vi "AuMT8852B EDR Rel Outp Pwr Summary Test.vi"() -> ()   [LabVIEW 2017]
doc: "This example shows how to extract Summary Test Results from the instrument. The Results panel will show a measurement summary of the test run. To view results from invividual test stages, use the Extended Test VIs."
panel:
  out "Results":T1 {"Peak 2DHx DPSK Absolute Power (dBm)" format="%.2f"; "Avg 2DHx DPSK Absolute Power (dBm)" format="%.2f"; "Min 2DHx DPSK Absolute Power (dBm)" format="%.2f"; "Max 2DHx DPSK Absolute Power (dBm)" format="%.2f"; "Peak 2DHx GFSK Absolute Power (dBm)" format="%.2f"; "Avg 2DHx GFSK Absolute Power (dBm)" format="%.2f"; "Min 2DHx GFSK Absolute Power (dBm)" format="%.2f"; "Max 2DHx GFSK Absolute Power (dBm)" format="%.2f"; "Peak 3DHx DPSK Absolute Power (dBm)" format="%.2f"; "Avg 3DHx DPSK Absolute Power (dBm)" format="%.2f"; "Min 3DHx DPSK Absolute Power (dBm)" format="%.2f"; "Max 3DHx DPSK Absolute Power (dBm)" format="%.2f"; "Peak 3DHx GFSK Absolute Power (dBm)" format="%.2f"; "Avg 3DHx GFSK Absolute Power (dBm)" format="%.2f"; "Min 3DHx GFSK Absolute Power (dBm)" format="%.2f"; "Max 3DHx GFSK Absolute Power (dBm)" format="%.2f"; "Avg power difference (dBm)" format="%.2f"; "Min power difference (dBm)" format="%.2f"; "Max power difference (dBm)" format="%.2f"; "Avg power difference (dBm)" format="%.2f"; "Min power difference (dBm)" format="%.2f"; "Max power difference (dBm)" format="%.2f"}
  in  "Settings":T2={"Low frequency selection"=enum."Use low frequency", "Medium frequency selection"=enum."Use medium frequency", "High frequency selection"=enum."Use high frequency", "Low TX frequency"=2480.0, "Low RX frequency"=2402.0, "Medium TX frequency"=2402.0, "Medium RX frequency"=2441.0, "High TX frequency"=2402.0, "High RX frequency"=2480.0, "Number of packets"=10, "PDPSK-PGFSK upper limit (dB) "=1.0, "PDPSK-PGFSK lower limit (dB)"=4.0, "2DHx test packet"=enum."Longest", "3DHx test packet"=enum."Longest", "Hop selection"=enum."Test with hopping off", "Test control"=enum."Loopback", "Hop mode"=enum."Defined", "Output Power Level"=enum."Max & Min"} {"PDPSK-PGFSK lower limit (dB)" format="%.2f"; "PDPSK-PGFSK upper limit (dB)" format="%.2f"}
  out "Addresses":string[](array[string])
  in  "Start/Stop (Start)":enum16{"Start", "Stop"}(ring)
  out "error out":errorcluster
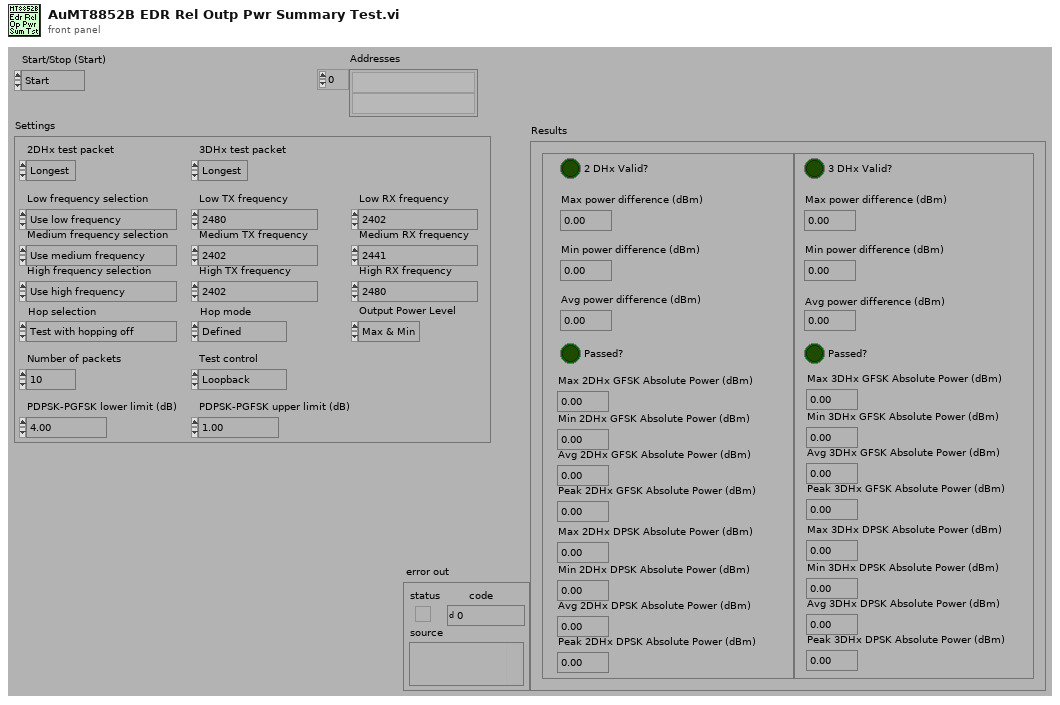
[diagram p1: front panel]
types:
  T1 = cluster{"2 DHx Valid?":bool, "Max power difference (dBm)":dbl, "Min power difference (dBm)":dbl, "Avg power difference (dBm)":dbl, "Passed?":bool, "3 DHx Valid?":bool, "Max power difference (dBm)":dbl, "Min power difference (dBm)":dbl, "Avg power difference (dBm)":dbl, "Passed?":bool, "Max 3DHx GFSK Absolute Power (dBm)":dbl, "Min 3DHx GFSK Absolute Power (dBm)":dbl, "Avg 3DHx GFSK Absolute Power (dBm)":dbl, "Peak 3DHx GFSK Absolute Power (dBm)":dbl, "Max 3DHx DPSK Absolute Power (dBm)":dbl, "Min 3DHx DPSK Absolute Power (dBm)":dbl, "Avg 3DHx DPSK Absolute Power (dBm)":dbl, "Peak 3DHx DPSK Absolute Power (dBm)":dbl, "Max 2DHx GFSK Absolute Power (dBm)":dbl, "Min 2DHx GFSK Absolute Power (dBm)":dbl, "Avg 2DHx GFSK Absolute Power (dBm)":dbl, "Peak 2DHx GFSK Absolute Power (dBm)":dbl, "Max 2DHx DPSK Absolute Power (dBm)":dbl, "Min 2DHx DPSK Absolute Power (dBm)":dbl, "Avg 2DHx DPSK Absolute Power (dBm)":dbl, "Peak 2DHx DPSK Absolute Power (dBm)":dbl}
  T2 = cluster{"Low frequency selection":enum16{"Don't use low frequency", "Use low frequency"}, "Medium frequency selection":enum16{"Don't use medium frequency", "Use medium frequency"}, "High frequency selection":enum16{"Don't use high frequency", "Use high frequency"}, "Low TX frequency":dbl, "Low RX frequency":dbl, "Medium TX frequency":dbl, "Medium RX frequency":dbl, "High TX frequency":dbl, "High RX frequency":dbl, "Number of packets":i32, "PDPSK-PGFSK upper limit (dB) ":dbl, "PDPSK-PGFSK lower limit (dB)":dbl, "2DHx test packet":enum16{"OFF", "Longest", "2-DH1", "2-DH3", "2-DH5"}, "3DHx test packet":enum16{"OFF", "Longest", "3-DH1", "3-DH3", "3-DH5"}, "Hop selection":enum16{"Test with hopping on", "Test with hopping off", "Test with hopping off and on"}, "Test control":enum16{"Loopback", "TX test"}, "Hop mode":enum16{"All", "Any", "Defined"}, "Output Power Level":enum16{"Min only", "Max only", "Max & Min"}}
  T3 = cluster{"Event status":enum16{"Event status disabled", "Event status enabled"}, "Message":enum16{"Message available disabled", "Message available enabled"}, "EUT Power State":u16, "State change":enum16{"State change disabled", "State change enabled"}, "Test failure":enum16{"Test failure disabled", "Test failure enabled"}, "Instrument status":enum16{"Instrument status disabled", "Instrument status enabled"}}
  T4 = cluster{"Completion":enum16{"Completion event disabled", "Completion event enabled"}, "Disconnect":enum16{"Disconnect event disabled", "Disconnect event enabled"}, "Connect":enum16{"Connect event disabled", "Connect event enabled"}, "Inquiry":enum16{"Inquiry event disabled", "Inquiry event enabled"}, "Temperature":enum16{"Temperature warning disabled", "Temperature warning enabled"}}
  T5 = cluster{"Reset":enum16{"Don't reset", "Reset"}, "Identity checking":enum16{"Don't query identity", "Query identity"}, "Simulation":enum16{"Don't simulate", "Simulate"}, "Range checking":enum16{"Don't check attribute ranges", "Check attribute ranges"}, "State caching":enum16{"Don't cache attributes", "Cache attributes"}, "Status checking":enum16{"Don't query instrument status", "Query instrument status"}}
  T6 = cluster{"Output power (Selected)":enum16{"Output power not selected", "Output power selected"}, "Power control (Selected)":enum16{"Power control not selected", "Power control selected"}, "Modulation index (Selected)":enum16{"Modulation index not selected", "Modulation index selected"}, "Initial carrier (Selected)":enum16{"Initial carrier not selected", "Initial carrier selected"}, "Carrier drift (Selected)":enum16{"Carrier drift not selected", "Carrier drift selected"}, "Single-slot sensitivity (Selected)":enum16{"Single-slot sensitivity not selected", "Single-slot sensitivity selected"}, "Multi-slot sensitivity (Selected)":enum16{"Multi-slot sensitivity not selected", "Multi-slot sensitivity selected"}, "Maximum input power (Selected)":enum16{"Maximum input power not selected", "Maximum input power selected"}, "Relative transmit power (Selected)":enum16{"Rel. transmit power not selected", "Rel. transmit power selected"}, "Carrier frequency stability and modulation (Selected)":enum16{"Carrier freq. and stability not selected", "Carrier freq. and stability selected"}, "Differential phase encoding":enum16{"Differential phase not selected", "Differential phase selected"}, "Sensitivity (Selected)":enum16{"Sensitivity not selected", "Sensitivity selected"}, "BER floor sensitivity (Selected)":enum16{"BER floor sensitivity not selected", "BER floor sensitivity selected"}, "EDR Maximum input power (Selected)":enum16{"EDR Max input power not selected", "EDR Max input power selected"}}
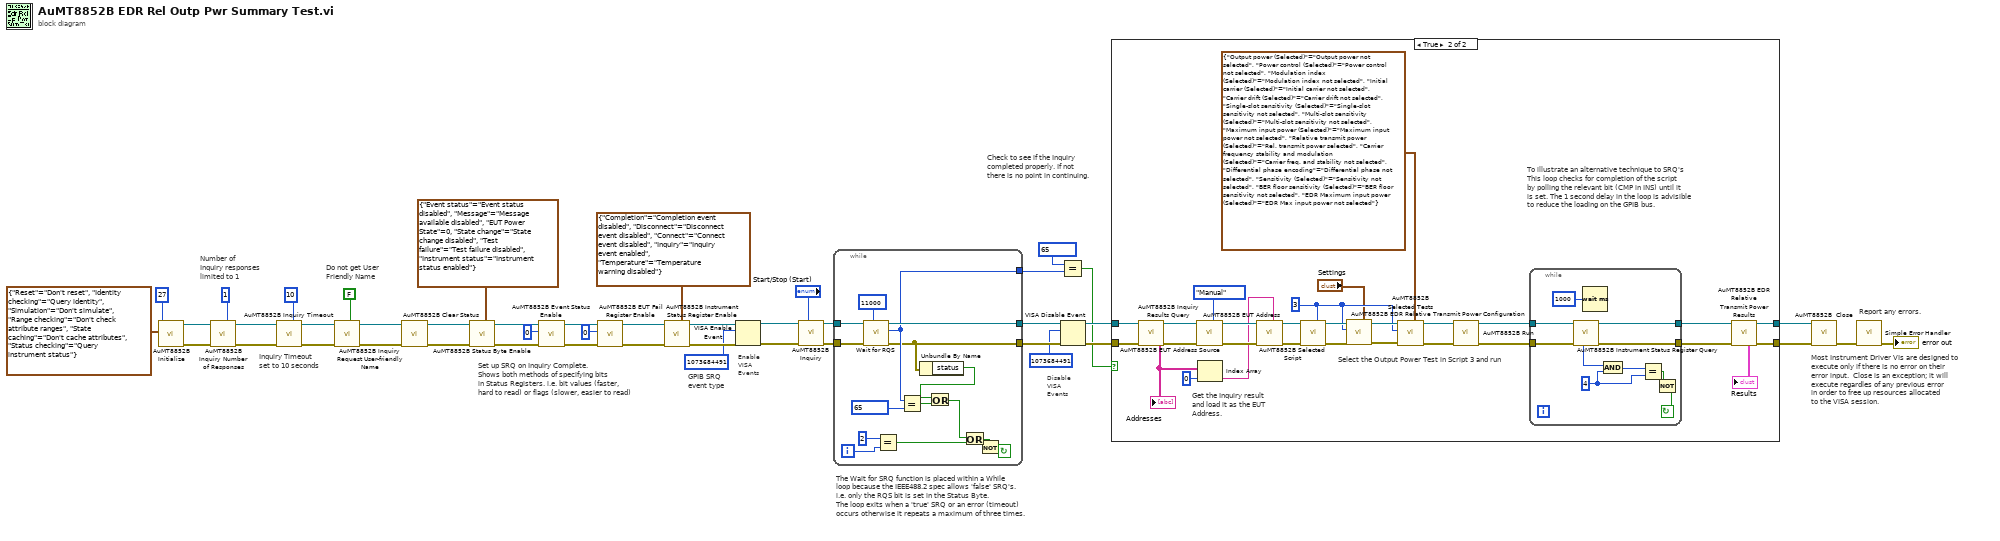
[diagram p0: block diagram]
diagram:
  # "Most Instrument Driver VIs are designed to\nexecute only if there is no error on their\nerror input.  Close is an exception; it will \nexecute regardles of any previous error\nin order to free up resources allocated\nto the VISA session."
  # "Report any errors."
  # "Check to see if the Inquiry\ncompleted properly. If not\nthere is no point in continuing."
  # "Disable\nVISA\nEvents"
  # "The Wait for SRQ function is placed within a While\nloop because the IEEE488.2 spec allows 'false' SRQ's.\ni.e. only the RQS bit is set in the Status Byte.\nThe loop exits when a 'true' SRQ or an error (timeout) \noccurs otherwise it repeats a maximum of three times."
  # "Enable\nVISA\nEvents"
  # "Set up SRQ on Inquiry Complete.\nShows both methods of specifying bits\nin Status Registers. i.e. bit values (faster, \nhard to read) or flags (slower, easier to read)"
  # "Inquiry Timeout\nset to 10 seconds"
  # "Number of\nInquiry responses\nlimited to 1"
  # "GPIB SRQ\nevent type"
  # "Do not get User\nFriendly Name"
  n1 = call <instrlib>:"AuMT8852B  Initialize.vi"("Options"=T5 {"Reset"=enum."Don't reset", "Identity checking"=enum."Query identity", "Simulation"=enum."Don't simulate", "Range checking"=enum."Don't check attribute ranges", "State caching"=enum."Don't cache attributes", "Status checking"=enum."Query instrument status"}, "GPIB Address (27)"=27) -> ("error out"=w43:errorcluster, "VISA session out"=w44:refnum<visa-resource-name>)  [unwired: 8 in]
  n2 = call <instrlib>:"AuMT8852B Inquiry Number of Responses.vi"("Responses (1)"=1, "error in (no error)"=w43, "VISA session"=w44) -> ("error out"=w41:errorcluster, "VISA session out"=w42:refnum<visa-resource-name>)  [unwired: 5 in, 2 out]
  n3 = call <instrlib>:"AuMT8852B Inquiry Timeout.vi"("Timeout (1)"=10, "error in (no error)"=w41, "VISA session"=w42) -> ("error out"=w38:errorcluster, "VISA session out"=w39:refnum<visa-resource-name>)  [unwired: 5 in, 2 out]
  n4 = call <instrlib>:"AuMT8852B Inquiry Request User-friendly Name.vi"("Status (T)"=FALSE, "error in (no error)"=w38, "VISA session"=w39) -> ("error out"=w33:errorcluster, "VISA session out"=w34:refnum<visa-resource-name>)  [unwired: 5 in, 2 out]
  n5 = call <instrlib>:"AuMT8852B Clear Status.vi"("error in (no error)"=w33, "VISA session"=w34) -> ("error out"=w31:errorcluster, "VISA session out"=w32:refnum<visa-resource-name>)  [unwired: 7 in, 1 out]
  n6 = call <instrlib>:"AuMT8852B Status Byte Enable.vi"("Flags in (all disabled)"=T3 {"Event status"=enum."Event status disabled", "Message"=enum."Message available disabled", "EUT Power State"=0, "State change"=enum."State change disabled", "Test failure"=enum."Test failure disabled", "Instrument status"=enum."Instrument status enabled"}, "error in (no error)"=w31, "VISA session"=w32) -> ("error out"=w30:errorcluster, "VISA session out"=w27:refnum<visa-resource-name>)  [unwired: 4 in, 3 out]
  n7 = call <instrlib>:"AuMT8852B Event Status Enable.vi"("error in (no error)"=w30, "Value (-1)"=0, "VISA session"=w27) -> ("error out"=w29:errorcluster, "VISA session out"=w26:refnum<visa-resource-name>)  [unwired: 4 in, 3 out]
  n8 = call <instrlib>:"AuMT8852B EUT Fail Register Enable.vi"("error in (no error)"=w29, "Value (-1)"=0, "VISA session"=w26) -> ("error out"=w28:errorcluster, "VISA session out"=w25:refnum<visa-resource-name>)  [unwired: 4 in, 3 out]
  n9 = call <instrlib>:"AuMT8852B Instrument Status Register Enable.vi"("Flags"=T4 {"Completion"=enum."Completion event disabled", "Disconnect"=enum."Disconnect event disabled", "Connect"=enum."Connect event disabled", "Inquiry"=enum."Inquiry event enabled", "Temperature"=enum."Temperature warning disabled"}, "error in (no error)"=w28, "VISA session"=w25) -> ("error out"=w20:errorcluster, "VISA session out"=w21:refnum<visa-resource-name>)  [unwired: 4 in, 3 out]
  n10 = VISA Enable Event(8:w20, 10:u32 1073684491 ("event type"), 11:w21) -> (0:w18:errorcluster, 3:w19:refnum<visa-resource-name>)  [unwired: 1 in]
  n11 = call <instrlib>:"AuMT8852B Inquiry.vi"("Start/Stop (Start)"="Start/Stop (Start)", "error in (no error)"=w18, "VISA session"=w19) -> ("error out"=w16:errorcluster, "VISA session out"=w17:refnum<visa-resource-name>)  [unwired: 6 in, 1 out]
  n12 = while {
    tunnel: w17 -> [w60]
    tunnel: w16 -> [w59]
    tunnel: [w58] -> w15
    tunnel: [w50] -> w14
    tunnel: [w51] -> w8
    i -> [w55]
    stop <- w46 continue-if-true
    n13 = call <vilib>:"Wait for RQS.VI"("timeout (25000 ms)"=u32 11000 ("timeout ms"), "error in (no error)"=w59, "VISA resource name"=w60) -> ("error out"=w50:errorcluster, "status byte"=w51:u16, "VISA resource name out"=w58:refnum<visa-resource-name>)  [unwired: 6 in]
    n14 = Equal?(x=2, y=w55) -> (x = y?=w56:bool)
    n15 = Equal?(x=w51, y=u16 65) -> (x = y?=w49:bool)
    n16 = Unbundle By Name(w50) -> ("status"=w48:bool)
    n17 = Or(x=w48, y=w49) -> (x .or. y?=w47:bool)
    n18 = Or(x=w47, y=w56) -> (x .or. y?=w57:bool)
    n19 = Not(x=w57) -> (.not. x?=w46:bool)
  }
  n20 = Equal?(x=u16 65, y=w8) -> (x = y?=w9:bool)
  n21 = VISA Disable Event(8:w14, 10:u32 1073684491 ("event type"), 11:w15) -> (0:w12:errorcluster, 3:w13:refnum<visa-resource-name>)  [unwired: 1 in]
  n22 = case shown="True" w9 {
    tunnel: [w62 w78] -> w40
    tunnel: w13 -> [w62 w90]
    tunnel: w12 -> [w61 w89]
    tunnel: [w61 w75] -> w4
    frame False {
    }
    frame True {
      w65 = 3 ("Script (3)")
      # "To illustrate an alternative technique to SRQ's\nThis loop checks for completion of the script\nby polling the relevant bit (CMP in INS) until it\nis set. The 1 second delay in the loop is advisible\nto reduce the loading on the GPIB bus."
      # "Select the Output Power Test in Script 3 and run"
      # "Get the Inquiry result\nand load it as the EUT\nAddress."
      n23 = call <instrlib>:"AuMT8852B Inquiry Results Query.vi"("error in (no error)"=w89, "VISA session"=w90) -> ("error out"=w87:errorcluster, "VISA session out"=w88:refnum<visa-resource-name>, "Addresses"=w83:string[])  [unwired: 5 in, 2 out]
      "Addresses" <- w83
      n24 = call <instrlib>:"AuMT8852B EUT Address Source.vi"("Source (Manual)"=enum16{"Manual", "RS-232", "USB", "Inquiry"}."Manual", "error in (no error)"=w87, "VISA session"=w88) -> ("error out"=w85:errorcluster, "VISA session out"=w84:refnum<visa-resource-name>)  [unwired: 5 in, 2 out]
      n25 = Index Array(array=w83, index=0 ("Index")) -> (element=w81:string)
      n26 = call <instrlib>:"AuMT8852B EUT Address.vi"("EUT Address (0x000000000000)"=w81, "error in (no error)"=w85, "VISA session"=w84) -> ("error out"=w77:errorcluster, "VISA session out"=w80:refnum<visa-resource-name>)  [unwired: 5 in, 2 out]
      n27 = call <instrlib>:"AuMT8852B Selected Script.vi"("Script (3)"=w65, "error in (no error)"=w77, "VISA session"=w80) -> ("error out"=w69:errorcluster, "VISA session out"=w67:refnum<visa-resource-name>)  [unwired: 5 in, 2 out]
      n28 = call <instrlib>:"AuMT8852B EDR Relative Transmit Power Configuration.vi"("Settings"="Settings", "error in (no error)"=w69, "Script (3)"=w65, "VISA session"=w67) -> ("error out"=w68:errorcluster, "VISA session out"=w66:refnum<visa-resource-name>)  [unwired: 4 in, 2 out]
      n29 = call <instrlib>:"AuMT8852B Selected Tests.vi"("Tests (All selected)"=T6 {"Output power (Selected)"=enum."Output power not selected", "Power control (Selected)"=enum."Power control not selected", "Modulation index (Selected)"=enum."Modulation index not selected", "Initial carrier (Selected)"=enum."Initial carrier not selected", "Carrier drift (Selected)"=enum."Carrier drift not selected", "Single-slot sensitivity (Selected)"=enum."Single-slot sensitivity not selected", "Multi-slot sensitivity (Selected)"=enum."Multi-slot sensitivity not selected", "Maximum input power (Selected)"=enum."Maximum input power not selected", "Relative transmit power (Selected)"=enum."Rel. transmit power selected", "Carrier frequency stability and modulation (Selected)"=enum."Carrier freq. and stability not selected", "Differential phase encoding"=enum."Differential phase not selected", "Sensitivity (Selected)"=enum."Sensitivity not selected", "BER floor sensitivity (Selected)"=enum."BER floor sensitivity not selected", "EDR Maximum input power (Selected)"=enum."EDR Max input power not selected"}, "error in (no error)"=w68, "Script (3)"=w65, "VISA session"=w66) -> ("error out"=w76:errorcluster, "VISA session out"=w79:refnum<visa-resource-name>)  [unwired: 4 in, 2 out]
      n30 = call <instrlib>:"AuMT8852B Run.vi"("error in (no error)"=w76, "VISA session"=w79) -> ("error out"=w72:errorcluster, "VISA session out"=w74:refnum<visa-resource-name>)  [unwired: 7 in, 1 out]
      n31 = while {
        tunnel: w74 -> [w100]
        tunnel: [w99] -> w73
        tunnel: w72 -> [w98]
        tunnel: [w97] -> w71
        stop <- w91 continue-if-true
        w92 = 4 ("y")
        n32 = call <instrlib>:"AuMT8852B Instrument Status Register Query.vi"("error in (no error)"=w98, "VISA session"=w100) -> ("error out"=w97:errorcluster, "VISA session out"=w99:refnum<visa-resource-name>, "Value"=w93:i32)  [unwired: 5 in, 2 out]
        n33 = Wait (ms)(milliseconds to wait=u32 1000) -> ()  [unwired: 1 out]
        n34 = And(x=w93, y=w92) -> (x .and. y?=w94:i32)
        n35 = Equal?(x=w94, y=w92) -> (x = y?=w95:bool)
        n36 = Not(x=w95) -> (.not. x?=w91:bool)
      }
      n37 = call <instrlib>:"AuMT8852B EDR Relative Transmit Power Results.vi"("error in (no error)"=w71, "VISA session"=w73) -> ("error out"=w75:errorcluster, "VISA session out"=w78:refnum<visa-resource-name>, "Results"=→"Results":T1)  [unwired: 6 in, 1 out]
    }
  }
  n38 = call <instrlib>:"AuMT8852B  Close.vi"("error in (no error)"=w4, "VISA session"=w40) -> ("error out"=w2:errorcluster)  [unwired: 8 in, 1 out]
  n39 = call <vilib>:"Simple Error Handler.vi"("error in (no error)"=w2) -> ("error out"=→"error out":errorcluster)  [unwired: 4 in, 4 out]
